vi "setLogicInChannel.vi"(7 "inputTypeStr":string, 8 "error in (no error)":errorcluster, 9 "sensitivtyStr":string, 11 "pHandle":u32) -> (0 "error out":errorcluster, 3 "return type":i32)   [LabVIEW 2011, in "sbgLabView.lvlib"]
uses:
  sbgLabView.lvlib
  sbgMatLab.dll
panel:
  in  "nsDelay":i32
  in  "locationStr":string
  in  "channel":u8
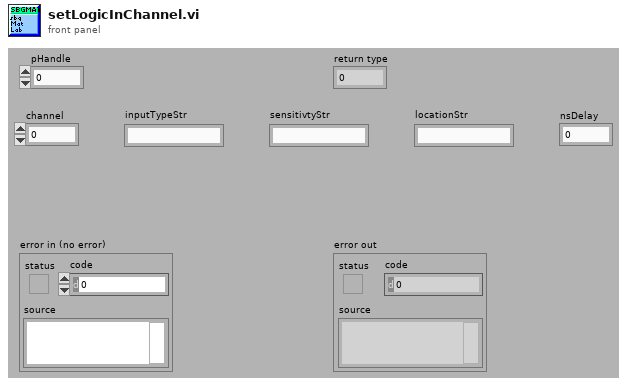
[diagram p1: front panel]
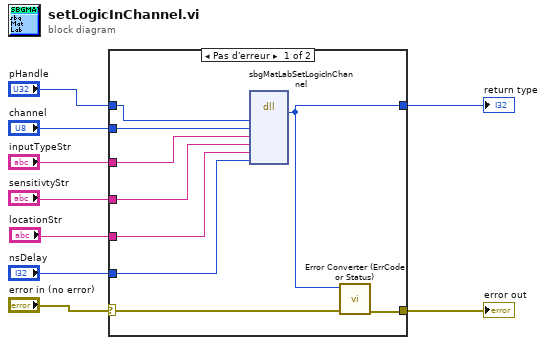
[diagram p0: block diagram]
diagram:
  n1 = case shown="Pas d'erreur" "error in (no error)" {
    selector: "error in (no error)" -> [w16 w19]
    tunnel: [w15 w19] -> w8
    tunnel: [w18 _] -> w7
    tunnel: "pHandle" -> [w17 _]
    tunnel: "channel" -> [w14 _]
    tunnel: "inputTypeStr" -> [w13 _]
    tunnel: "sensitivtyStr" -> [w12 _]
    tunnel: "locationStr" -> [w11 _]
    tunnel: "nsDelay" -> [w10 _]
    frame No Error {
      n2 = dll-call lib="C:/SBG-Systems/remote/projects/software/projects/labviewExample/sbgLabView/sbgMatLab.*" fn="sbgMatLabSetLogicInChannel" ("sbgMatLab.dll:sbgMatLabSetGpsOptions")("pHandle"=w17, "channel"=w14, "inputTypeStr"=w13, "sensitivityStr"=w12, "locationStr"=w11, "nsDelay"=w10) -> ("return type"=w18:i32)  [unwired: 9 in, 2 out]
      n3 = call "Error Converter (ErrCode or Status).vi"("error in (no error)"=w16, "error code"=w18) -> ("error out"=w15:errorcluster)  [unwired: 9 in]
    }
    frame Error {
    }
  }
  "return type" <- w7
  "error out" <- w8
